vi "Read Teardown Init.vi"(11 "Actor in":refnum<class "Actor.lvclass">) -> (2 "Teardown Init":bool)   [LabVIEW 2020, in "jettl.lvlib" / "Actor.lvlib" / "Actor.lvclass"]
uses:
  Actor.lvclass
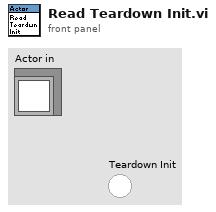
[diagram p1: front panel]
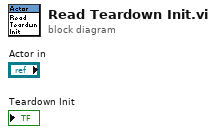
[diagram p0: block diagram]
diagram:
